vi "PRIME Gen Filenames.vi"(9 "Observation":T1={"Priority"=0, "ID"="", "Observer"="", "Obj Name"="", "Obj Type"="", "RA and DEC String"={"RA"="HH:MM:SS.nnn", "DEC"="DEG:arcmin:arcsec.nn"}, "Filter Wheel 1"="", "Filter Wheel 2"="", "Integration Time"=0.0, "Observation Status"=enum."Error", "Offsets"={"RA"=0.0, "DEC"=0.0, "ROT"=0.0}, "Images"=0, "Dither Options"={"Dither"=enum."None", "Dither Radius"=0.0, "Dither Points"=0, "Dither Phase"=0.0}, "Comment 1"="", "Comment 2"=""}, 10 "Detector Config":T7={"Detector"=0, "Offsets"=[[0, 0, 0, 0, 0, 0, 0, 0, 0, 0, 0, 0, 0, 0, 0, 0, 0, 0, 0, 0, 0, 0, 0, 0, 0, 0, 0, 0, 0, 0, 0, 0]], "Detector Computer"={"Machine"="192.168.121.11", "Password"="rSL!nux23456", "FITS File Path"="", "Port"=44444, "Header Path"="", "Name"=""}, "FITS hdr template0"=path "", "FITS hdr template1"=path "", "FITS Data File Path"=path "", "FITS Detector Settings"={"Exp Time Short"=0.0, "# of Frames"=0.0, "Exp Time Long"=0.0, "# of Groups"=0.0, "Object Name"="", "Object"="", "Obs Type"="", "Image Type"="", "Observer"="", "Observer Affiliation"=""}, "Sim Folder"=path "", "Integration Mode"=enum."SSR", "Integration Time"=0.0, "Frame Int Time"=0.0} {"Offsets" format="%04x"; "Detector" items=["0", "1", "2"]}, 11 "Raw Files":T6) -> (0 "Exp Count out":i32, 1 "Source Files":path[](array[path]), 2 "Filenames":string[](array[string]), 3 "Table":string[](array[string]))   [LabVIEW 2021]
uses:
  RIMAS Detector Config.ctl
  RIMAS Detector Server Config.ctl
  RIMAS Observation Config.ctl
  Detector enum Detector Integration Mode.ctl
  Detector cluster Files.ctl
  typedefs/CC cluster Observation.ctl
  Observation Queue/CC enum Observation Status.ctl
  Telescope/CC cluster Telescope Offsets.ctl
  typedefs/CC cluster Observation Dither Options.ctl
  typedefs/CC enum Dither Selection.ctl
  PRIME Detector cluster Status.ctl
  FITS/PRIME cluster File Counter.ctl
  Logging/CC enum Current Values Action.ctl
  hk-channel-class/HK Table/HK Table.lvclass
  Detector Class.lvclass
panel:
  # "sec"
  # "sec"
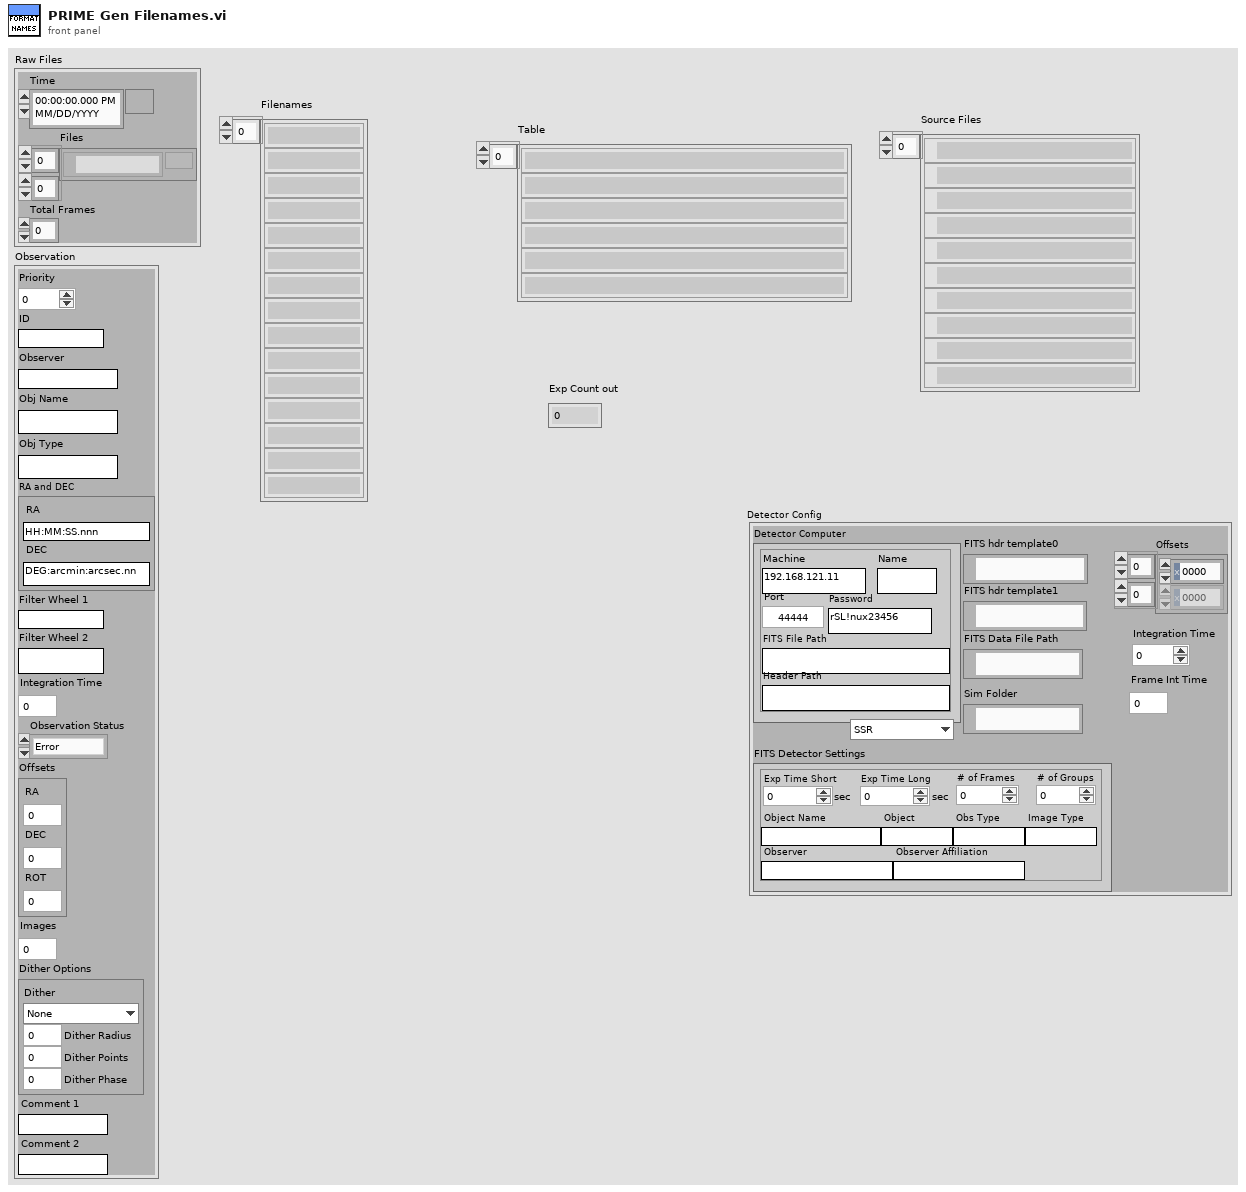
[diagram p1: front panel]
types:
  T1 = typedef "CC cluster Observation.ctl" = cluster{"Priority":i32, "ID":string, "Observer":string, "Obj Name":string, "Obj Type":string, "RA and DEC String":cluster{"RA":string, "DEC":string}, "Filter Wheel 1":string, "Filter Wheel 2":string, "Integration Time":dbl, "Observation Status":T2, "Offsets":T3, "Images":i32, "Dither Options":T4, "Comment 1":string, "Comment 2":string}
  T2 = typedef "CC enum Observation Status.ctl" = enum16{"Ready", "Running", "Done", "Error"}
  T3 = typedef "CC cluster Telescope Offsets.ctl" = cluster{"RA":dbl, "DEC":dbl, "ROT":dbl}
  T4 = typedef "CC cluster Observation Dither Options.ctl" = cluster{"Dither":T5, "Dither Radius":dbl, "Dither Points":i32, "Dither Phase":dbl}
  T5 = typedef "CC enum Dither Selection.ctl" = enum16{"None", "Circle", "Random"}
  T6 = typedef "Detector Class.lvclass/Detector cluster Files.ctl" = cluster{"Time":timestamp, "Files":path[][], "Total Frames":i32}
  T7 = typedef "RIMAS Detector Config.ctl" = cluster{"Detector":u16, "Offsets":u16[][], "Detector Computer":T8, "FITS hdr template0":path, "FITS hdr template1":path, "FITS Data File Path":path, "FITS Detector Settings":T9, "Sim Folder":path, "Integration Mode":T10, "Integration Time":dbl, "Frame Int Time":dbl}
  T8 = typedef "RIMAS Detector Server Config.ctl" = cluster{"Machine":string, "Password":string, "FITS File Path":string, "Port":u16, "Header Path":string, "Name":string}
  T9 = typedef "RIMAS Observation Config.ctl" = cluster{"Exp Time Short":dbl, "# of Frames":dbl, "Exp Time Long":dbl, "# of Groups":dbl, "Object Name":string, "Object":string, "Obs Type":string, "Image Type":string, "Observer":string, "Observer Affiliation":string}
  T10 = typedef "Detector enum Detector Integration Mode.ctl" = enum16{"SSR", "CDS", "MEAN", "MEDIAN", "MODE", "MIIN", "MAX"}
  T11 = typedef "CC enum Current Values Action.ctl" = enum16{"Init", "Write Item", "Write Array", "Read Item", "Read Array", "Read All", "Add Channels", "New File", "Add Message", "Get Current Values", "Close"}
  T12 = typedef "PRIME cluster File Counter.ctl" = cluster{"File Count":i32}
  T13 = typedef "PRIME Detector cluster Status.ctl" = cluster{"Cmd Start Time":timestamp, "Command":string, "Complete?":bool, "Cmd Complete Time":timestamp, "Exp Time Remaining":dbl, "Total Frames":i32, "Exp Frames":cluster{"CAMERA0":string[], "CAMERA1":string[], "CAMERA2":string[], "CAMERA3":string[]}, "Intermediate Frames":cluster{"CAMERA0":string[], "CAMERA1":string[], "CAMERA2":string[], "CAMERA3":string[]}, "Final Reduced Frame":cluster{"CAMERA0":string, "CAMERA1":string, "CAMERA2":string, "CAMERA3":string}}
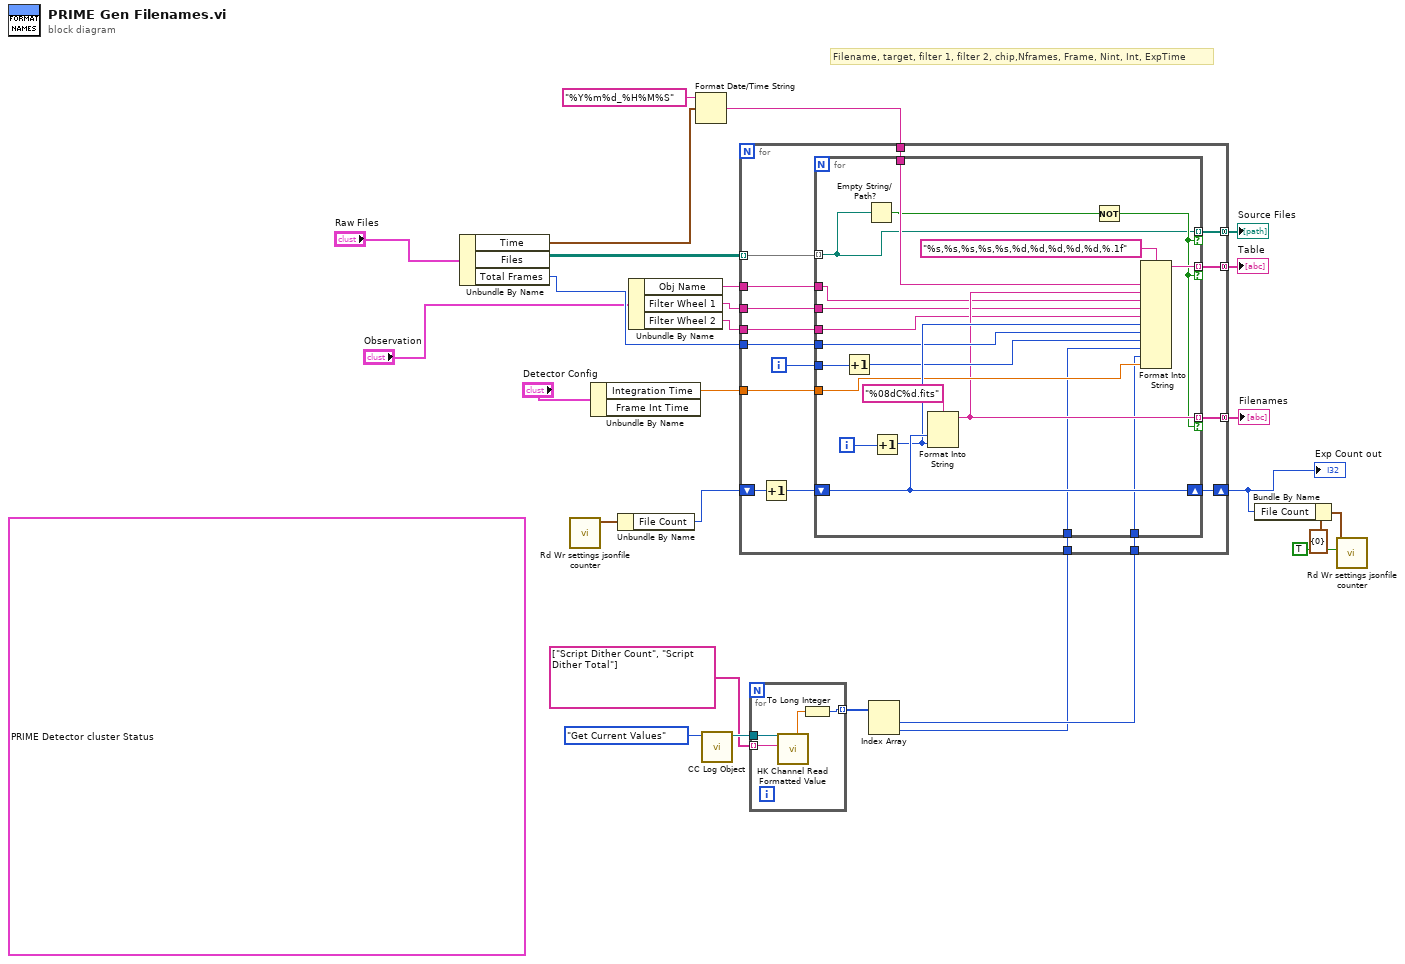
[diagram p0: block diagram]
diagram:
  (unwired) T13 {"Cmd Start Time"=timestamp(3729599083.065959 s since 1904-01-01), "Command"="START", "Complete?"=TRUE, "Cmd Complete Time"=timestamp(3729599162.21691 s since 1904-01-01), "Exp Time Remaining"=0.0, "Total Frames"=8, "Exp Frames"={"CAMERA0"=["C:\\Users\\gsfcprime\\PycharmProjects\\asdetector\\output\\raw\\20220308\\prime.0000.C0\\prime.0000.C0.000000.fits", "C:\\Users\\gsfcprime\\PycharmProjects\\asdetector\\output\\raw\\20220308\\prime.0000.C0\\prime.0000.C0.000001.fits", "C:\\Users\\gsfcprime\\PycharmProjects\\asdetector\\output\\raw\\20220308\\prime.0000.C0\\prime.0000.C0.000002.fits", "C:\\Users\\gsfcprime\\PycharmProjects\\asdetector\\output\\raw\\20220308\\prime.0000.C0\\prime.0000.C0.000003.fits", "C:\\Users\\gsfcprime\\PycharmProjects\\asdetector\\output\\raw\\20220308\\prime.0000.C0\\prime.0000.C0.000004.fits", "C:\\Users\\gsfcprime\\PycharmProjects\\asdetector\\output\\raw\\20220308\\prime.0000.C0\\prime.0000.C0.000005.fits", "C:\\Users\\gsfcprime\\PycharmProjects\\asdetector\\output\\raw\\20220308\\prime.0000.C0\\prime.0000.C0.000006.fits", "C:\\Users\\gsfcprime\\PycharmProjects\\asdetector\\output\\raw\\20220308\\prime.0000.C0\\prime.0000.C0.000007.fits"], "CAMERA1"=["C:\\Users\\gsfcprime\\PycharmProjects\\asdetector\\output\\raw\\20220308\\prime.0000.C1\\prime.0000.C1.000000.fits", "C:\\Users\\gsfcprime\\PycharmProjects\\asdetector\\output\\raw\\20220308\\prime.0000.C1\\prime.0000.C1.000001.fits", "C:\\Users\\gsfcprime\\PycharmProjects\\asdetector\\output\\raw\\20220308\\prime.0000.C1\\prime.0000.C1.000002.fits", "C:\\Users\\gsfcprime\\PycharmProjects\\asdetector\\output\\raw\\20220308\\prime.0000.C1\\prime.0000.C1.000003.fits", "C:\\Users\\gsfcprime\\PycharmProjects\\asdetector\\output\\raw\\20220308\\prime.0000.C1\\prime.0000.C1.000004.fits", "C:\\Users\\gsfcprime\\PycharmProjects\\asdetector\\output\\raw\\20220308\\prime.0000.C1\\prime.0000.C1.000005.fits", "C:\\Users\\gsfcprime\\PycharmProjects\\asdetector\\output\\raw\\20220308\\prime.0000.C1\\prime.0000.C1.000006.fits", "C:\\Users\\gsfcprime\\PycharmProjects\\asdetector\\output\\raw\\20220308\\prime.0000.C1\\prime.0000.C1.000007.fits"], "CAMERA2"=["C:\\Users\\gsfcprime\\PycharmProjects\\asdetector\\output\\raw\\20220308\\prime.0000.C2\\prime.0000.C2.000000.fits", "C:\\Users\\gsfcprime\\PycharmProjects\\asdetector\\output\\raw\\20220308\\prime.0000.C2\\prime.0000.C2.000001.fits", "C:\\Users\\gsfcprime\\PycharmProjects\\asdetector\\output\\raw\\20220308\\prime.0000.C2\\prime.0000.C2.000002.fits", "C:\\Users\\gsfcprime\\PycharmProjects\\asdetector\\output\\raw\\20220308\\prime.0000.C2\\prime.0000.C2.000003.fits", "C:\\Users\\gsfcprime\\PycharmProjects\\asdetector\\output\\raw\\20220308\\prime.0000.C2\\prime.0000.C2.000004.fits", "C:\\Users\\gsfcprime\\PycharmProjects\\asdetector\\output\\raw\\20220308\\prime.0000.C2\\prime.0000.C2.000005.fits", "C:\\Users\\gsfcprime\\PycharmProjects\\asdetector\\output\\raw\\20220308\\prime.0000.C2\\prime.0000.C2.000006.fits", "C:\\Users\\gsfcprime\\PycharmProjects\\asdetector\\output\\raw\\20220308\\prime.0000.C2\\prime.0000.C2.000007.fits"], "CAMERA3"=["C:\\Users\\gsfcprime\\PycharmProjects\\asdetector\\output\\raw\\20220308\\prime.0000.C3\\prime.0000.C3.000000.fits", "C:\\Users\\gsfcprime\\PycharmProjects\\asdetector\\output\\raw\\20220308\\prime.0000.C3\\prime.0000.C3.000001.fits", "C:\\Users\\gsfcprime\\PycharmProjects\\asdetector\\output\\raw\\20220308\\prime.0000.C3\\prime.0000.C3.000002.fits", "C:\\Users\\gsfcprime\\PycharmProjects\\asdetector\\output\\raw\\20220308\\prime.0000.C3\\prime.0000.C3.000003.fits", "C:\\Users\\gsfcprime\\PycharmProjects\\asdetector\\output\\raw\\20220308\\prime.0000.C3\\prime.0000.C3.000004.fits", "C:\\Users\\gsfcprime\\PycharmProjects\\asdetector\\output\\raw\\20220308\\prime.0000.C3\\prime.0000.C3.000005.fits", "C:\\Users\\gsfcprime\\PycharmProjects\\asdetector\\output\\raw\\20220308\\prime.0000.C3\\prime.0000.C3.000006.fits", "C:\\Users\\gsfcprime\\PycharmProjects\\asdetector\\output\\raw\\20220308\\prime.0000.C3\\prime.0000.C3.000007.fits"]}, "Intermediate Frames"={"CAMERA0"=["C:\\Users\\gsfcprime\\PycharmProjects\\asdetector\\output\\res\\20220308\\prime.0000.C0\\prime.0000.C0.000000.fits", "C:\\Users\\gsfcprime\\PycharmProjects\\asdetector\\output\\res\\20220308\\prime.0000.C0\\prime.0000.C0.000001.fits", "C:\\Users\\gsfcprime\\PycharmProjects\\asdetector\\output\\res\\20220308\\prime.0000.C0\\prime.0000.C0.000002.fits", "C:\\Users\\gsfcprime\\PycharmProjects\\asdetector\\output\\res\\20220308\\prime.0000.C0\\prime.0000.C0.000003.fits", "C:\\Users\\gsfcprime\\PycharmProjects\\asdetector\\output\\res\\20220308\\prime.0000.C0\\prime.0000.C0.000004.fits", "C:\\Users\\gsfcprime\\PycharmProjects\\asdetector\\output\\res\\20220308\\prime.0000.C0\\prime.0000.C0.000005.fits", "C:\\Users\\gsfcprime\\PycharmProjects\\asdetector\\output\\res\\20220308\\prime.0000.C0\\prime.0000.C0.000006.fits", "C:\\Users\\gsfcprime\\PycharmProjects\\asdetector\\output\\res\\20220308\\prime.0000.C0\\prime.0000.C0.000007.fits"], "CAMERA1"=["C:\\Users\\gsfcprime\\PycharmProjects\\asdetector\\output\\res\\20220308\\prime.0000.C1\\prime.0000.C1.000000.fits", "C:\\Users\\gsfcprime\\PycharmProjects\\asdetector\\output\\res\\20220308\\prime.0000.C1\\prime.0000.C1.000001.fits", "C:\\Users\\gsfcprime\\PycharmProjects\\asdetector\\output\\res\\20220308\\prime.0000.C1\\prime.0000.C1.000002.fits", "C:\\Users\\gsfcprime\\PycharmProjects\\asdetector\\output\\res\\20220308\\prime.0000.C1\\prime.0000.C1.000003.fits", "C:\\Users\\gsfcprime\\PycharmProjects\\asdetector\\output\\res\\20220308\\prime.0000.C1\\prime.0000.C1.000004.fits", "C:\\Users\\gsfcprime\\PycharmProjects\\asdetector\\output\\res\\20220308\\prime.0000.C1\\prime.0000.C1.000005.fits", "C:\\Users\\gsfcprime\\PycharmProjects\\asdetector\\output\\res\\20220308\\prime.0000.C1\\prime.0000.C1.000006.fits", "C:\\Users\\gsfcprime\\PycharmProjects\\asdetector\\output\\res\\20220308\\prime.0000.C1\\prime.0000.C1.000007.fits"], "CAMERA2"=["C:\\Users\\gsfcprime\\PycharmProjects\\asdetector\\output\\res\\20220308\\prime.0000.C2\\prime.0000.C2.000000.fits", "C:\\Users\\gsfcprime\\PycharmProjects\\asdetector\\output\\res\\20220308\\prime.0000.C2\\prime.0000.C2.000001.fits", "C:\\Users\\gsfcprime\\PycharmProjects\\asdetector\\output\\res\\20220308\\prime.0000.C2\\prime.0000.C2.000002.fits", "C:\\Users\\gsfcprime\\PycharmProjects\\asdetector\\output\\res\\20220308\\prime.0000.C2\\prime.0000.C2.000003.fits", "C:\\Users\\gsfcprime\\PycharmProjects\\asdetector\\output\\res\\20220308\\prime.0000.C2\\prime.0000.C2.000004.fits", "C:\\Users\\gsfcprime\\PycharmProjects\\asdetector\\output\\res\\20220308\\prime.0000.C2\\prime.0000.C2.000005.fits", "C:\\Users\\gsfcprime\\PycharmProjects\\asdetector\\output\\res\\20220308\\prime.0000.C2\\prime.0000.C2.000006.fits", "C:\\Users\\gsfcprime\\PycharmProjects\\asdetector\\output\\res\\20220308\\prime.0000.C2\\prime.0000.C2.000007.fits"], "CAMERA3"=["C:\\Users\\gsfcprime\\PycharmProjects\\asdetector\\output\\res\\20220308\\prime.0000.C3\\prime.0000.C3.000000.fits", "C:\\Users\\gsfcprime\\PycharmProjects\\asdetector\\output\\res\\20220308\\prime.0000.C3\\prime.0000.C3.000001.fits", "C:\\Users\\gsfcprime\\PycharmProjects\\asdetector\\output\\res\\20220308\\prime.0000.C3\\prime.0000.C3.000002.fits", "C:\\Users\\gsfcprime\\PycharmProjects\\asdetector\\output\\res\\20220308\\prime.0000.C3\\prime.0000.C3.000003.fits", "C:\\Users\\gsfcprime\\PycharmProjects\\asdetector\\output\\res\\20220308\\prime.0000.C3\\prime.0000.C3.000004.fits", "C:\\Users\\gsfcprime\\PycharmProjects\\asdetector\\output\\res\\20220308\\prime.0000.C3\\prime.0000.C3.000005.fits", "C:\\Users\\gsfcprime\\PycharmProjects\\asdetector\\output\\res\\20220308\\prime.0000.C3\\prime.0000.C3.000006.fits", "C:\\Users\\gsfcprime\\PycharmProjects\\asdetector\\output\\res\\20220308\\prime.0000.C3\\prime.0000.C3.000007.fits"]}, "Final Reduced Frame"={"CAMERA0"="C:\\Users\\gsfcprime\\PycharmProjects\\asdetector\\output\\reduced\\20220308\\prime.0000.C0.fits", "CAMERA1"="C:\\Users\\gsfcprime\\PycharmProjects\\asdetector\\output\\reduced\\20220308\\prime.0000.C1.fits", "CAMERA2"="C:\\Users\\gsfcprime\\PycharmProjects\\asdetector\\output\\reduced\\20220308\\prime.0000.C2.fits", "CAMERA3"="C:\\Users\\gsfcprime\\PycharmProjects\\asdetector\\output\\reduced\\20220308\\prime.0000.C3.fits"}} ("prime detector status")
  # "Filename, target, filter 1, filter 2, chip,Nframes, Frame, Nint, Int, ExpTime"
  n1 = Unbundle By Name("Raw Files") -> ("Time"=w7:timestamp, "Files"=w6:path[][], "Total Frames"=w5:i32)
  n2 = call "Rd Wr settings jsonfile counter.vi"() -> ("FileCounter"=w20:T12)  [unwired: 10 in, 1 out]
  n3 = Unbundle By Name("Detector Config") -> ("Integration Time"=w25:dbl)  [unwired: 1 out]
  n4 = Unbundle By Name(w20) -> ("File Count"=w19:i32)
  n5 = Unbundle By Name("Observation") -> ("Obj Name"=w1:string, "Filter Wheel 1"=w2:string, "Filter Wheel 2"=w3:string)
  n6 = Format Date/Time String(time format string (%c)="%Y%m%d_%H%M%S", seconds (now)=w7) -> (date/time string=w21:string)  [unwired: 1 in]
  n7 = call "CC Log Object.vi"("Action"=CC_enum_Current_Values_Action."Get Current Values") -> ("HK Channel out"=w13:refnum<class "HK Table.lvclass">)  [unwired: 8 in, 2 out]
  n8 = for {
    tunnel: w13 -> [w31]
    tunnel: string[] ["Script Dither Count", "Script Dither Total"] -> [w30] mode=indexing
    tunnel: [w28] -> w11 mode=indexing
    n9 = call-dynamic "HK Channel Read Formatted Value.vi"("Name"=w30, "HK Channel in"=w31) -> ("Value"=w29:dbl)  [unwired: 2 in, 7 out]
    n10 = To Long Integer(number=w29) -> (32bit integer=w28:i32)
  }
  n11 = Index Array(array=w11) -> (element #1=w10:i32, element #2=w9:i32)  [unwired: 2 in]
  n12 = for {
    shift-right: [w47] -> w17
    shift-left: w19 -> [w46]
    tunnel: w6 -> [w45] mode=indexing
    tunnel: [w43] -> w27 mode=concatenating
    tunnel: w5 -> [w42]
    tunnel: w10 -> [w40]
    tunnel: w25 -> [w39]
    tunnel: [w38] -> w24 mode=concatenating
    tunnel: [w37] -> w23 mode=concatenating
    tunnel: w21 -> [w36]
    tunnel: w9 -> [w35]
    tunnel: w3 -> [w34]
    tunnel: w2 -> [w33]
    tunnel: w1 -> [w32]
    i -> [w41]
    n13 = Increment(x=w46) -> (x+1=w44:i32)
    n14 = for {
      shift-right: [w66] -> w47
      shift-left: w44 -> [w66]
      tunnel: w45 -> [w51] mode=indexing
      tunnel: [w57] -> w43 mode=indexing if=w55
      tunnel: w42 -> [w62]
      tunnel: w41 -> [w61]
      tunnel: w40 -> [w53]
      tunnel: w39 -> [w59]
      tunnel: [w58] -> w38 mode=indexing if=w55
      tunnel: [w51] -> w37 mode=indexing if=w55
      tunnel: w36 -> [w56]
      tunnel: w35 -> [w52]
      tunnel: w34 -> [w50]
      tunnel: w33 -> [w49]
      tunnel: w32 -> [w48]
      i -> [w65]
      n15 = Increment(x=w61) -> (x+1=w60:i32)
      n16 = Empty String/Path?(string/path=w51) -> (empty?=w54:bool)
      n17 = Increment(x=w65) -> (x+1=w63:i32)
      n18 = Format Into String(format string="%08dC%d.fits", w66, w63) -> (resulting string=w57:string)  [unwired: 2 in, 1 out]
      n19 = Not(x=w54) -> (.not. x?=w55:bool)
      n20 = Format Into String(format string="%s,%s,%s,%s,%s,%d,%d,%d,%d,%d,%.1f", w56, w57, w48, w49, w50, w63, w62, w60, w52, w53, w59) -> (resulting string=w58:string)  [unwired: 2 in, 1 out]
    }
  }
  "Filenames" <- w27
  "Table" <- w24
  "Exp Count out" <- w17
  "Source Files" <- w23
  n21 = Bundle By Name(cluster=T12 {"File Count"=0}, "File Count"=w17) -> (w16:T12)
  n22 = call "Rd Wr settings jsonfile counter.vi"("Write? (F:Read)"=TRUE, "FileCounter"=w16) -> ()  [unwired: 8 in, 2 out]
